vi "Global 1 Base.vi"() -> ()   [LabVIEW 2022 SP3]
panel:
  in  "Numeric":i32
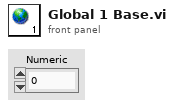
[diagram p1: front panel]
diagram:
